vi "Check and Override Channel Configuration.vi"(8 "error in (no error)":errorcluster, 10 "Custom Config Data in":u8[](array[numeric]) format="%.0x", 11 "CIFChannels in":refnum<class "CIFChannels.lvclass">) -> (0 "error out":errorcluster, 2 "Custom Config Data out":u8[](array[numeric]) format="%.0x", 3 "CIFChannels out":refnum<class "CIFChannels.lvclass">)   [LabVIEW 2021, in "CIFChannels.lvclass"]
uses:
  CIFChannels.lvclass
  ChannelCommon/typedef/Errors.ctl
  <vilib>/CIF Foundation/CIF Utilities/DataTypes/Unflatten U64.vi
  <vilib>/CIF Foundation/CIF Utilities/DataTypes/Flatten U64.vi
  <vilib>/CIF Foundation/CIF Utilities/Errors/Append Error Location.vi
  CIFChannels.lvclass/CIFChannels.ctl
  ChannelCommon/ChannelCommon.lvlib
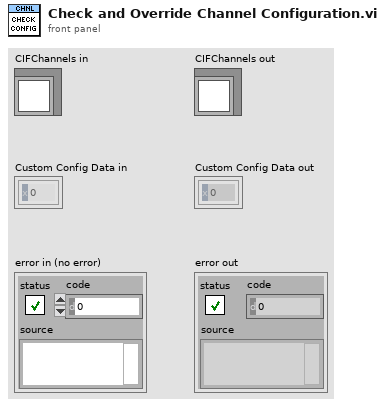
[diagram p1: front panel]
types:
  T1 = typedef "ChannelCommon.lvlib/Errors.ctl" = enum16{"gRPC Server Not Found", "Duplicate Channel", "Missing Channel", "Incorrect Type", "Flatten Error", "Unflatten Data", "Channel Length", "Plugin Connection", "gRPC Server Connection", "FIFO Unflatten", "Required Override"}
  T2 = typedef "ChannelCommon.lvlib/FIFO Config.ctl" = cluster{"Max Bytes/Msg":u64, "Max Msg/FIFO":u64, "Flags":u64}
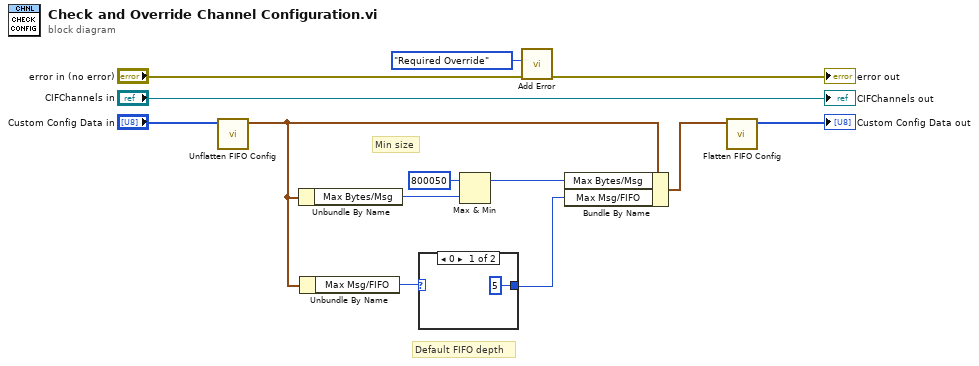
[diagram p0: block diagram]
diagram:
  # "Default FIFO depth"
  # "Min size"
  n1 = call "Unflatten FIFO Config.vi"("Flattened Data in"="Custom Config Data in") -> ("FIFO Config out"=w2:T2)  [unwired: 9 in, 1 out]
  n2 = Unbundle By Name(w2) -> ("Max Bytes/Msg"=w5:u64)
  n3 = Unbundle By Name(w2) -> ("Max Msg/FIFO"=w7:u64)
  n4 = case shown="0" w7 {
    selector: w7 -> [_ w15]
    tunnel: [u64 5 ("Max Msg/FIFO") w15] -> w6
    frame 0 {
    }
    frame 1, Default {
    }
  }
  n5 = Max & Min(x=u64 800050, y=w5) -> (max(x,y)=w4:u64)  [unwired: 1 out]
  n6 = call "Add Error.vi"("error in (no error)"="error in (no error)", "Error"=Errors."Required Override") -> ("error out"=→"error out":errorcluster)  [unwired: 9 in]
  n7 = Bundle By Name(cluster=w2, "Max Bytes/Msg"=w4, "Max Msg/FIFO"=w6) -> (w1:T2)
  n8 = call "Flatten FIFO Config.vi"("FIFO Config in"=w1) -> ("Flattened FIFO Config"=→"Custom Config Data out":u8[])  [unwired: 10 in]
  "CIFChannels out" <- "CIFChannels in"
